vi "RSZVB Set Virtual Transform Port Pair.vi"(0 "VISA session":refnum<visa-resource-name>, 1 "Parameter Type (Capacitance)":i32(ring) items=["Capacitance", "Inductance", "Resistance"], 2 "Circuit Model (Serial Touchstone (.s2p) data, shunt L)":i32(ring)=1 items=["Serial Touchstone (.s2p) data, shunt L"=1, "Serial Touchstone (.s2p) data, shunt C"=2, "Shunt L, serial Touchstone (.s2p) data"=3, "Shunt C, serial Touchstone (.s2p) data"=4, "Serial Cs, shunt L"=5, "Serial Ls, shunt C"=6, "Serial Cs, shunt C"=7, "Serial Ls, shunt L"=8, "Shunt L, serial Cs"=9, "Shunt C, serial Ls"=10, "Shunt C, serial Cs"=11, "Shunt L, serial Ls"=12], 5 "Channel (1)":i32=1, 7 "Function Type (Deembedding)":i32(ring) items=["Deembedding", "Embedding"], 9 "Port Pair (1)":i32=1, 11 "error in (no error)":errorcluster {"code" format="%.0x"}, 12 "Parameter Number (1)":i32=1, 13 "Value (1.0E-12)":dbl=1e-12 format="%^.3e") -> (4 "dup VISA session":refnum<visa-resource-name>, 15 "error out":errorcluster {"code" format="%.0x"})   [LabVIEW 2011]
doc: "This VI specifies the capacitance, inductance or resistance values C1, C2, C3, L1, L2, L3 or R1, R2, R3 in the different circuit models for port pair deembedding/embedding.\n\nRemote-control command(s):\nCALCulate<Ch>:TRANsform:VNETworks:PPAir:DEEMbedding<List_idx>:PARameters:C<no> STSC | SCST | CSSL | LSSC | CSSC | SLCS | SCLS | SCCS,<numeric_value>\nCALCulate<Ch>:TRANsform:VNETworks:PPAir:DEEMbedding<List_idx>:PARameters:L<no> STSL | SLST | CSSL | LSSC | LSSL | SLCS | SCLS | SLLS,<numeric_value>\nCALCulate<Ch>:TRANsform:VNETworks:PPAir:DEEMbedding<List_idx>:PARameters:R<no> STSL | STSC | SLST | SCST | CSSL | LSSC | CSSC | LSSL | SLCS | SCLS | SCCS | SLLS,<numeric_value>\nCALCulate<Ch>:TRANsform:VNETworks:PPAir:EMBedding<List_idx>:PARameters:C<no> STSC | SCST | CSSL | LSSC | CSSC | SLCS | SCLS | SCCS,<numeric_value>\nCALCulate<Ch>:TRANsform:VNETworks:PPAir:EMBedding<List_idx>:PARameters:L<no> STSL | SLST | CSSL | LSSC | LSSL | SLCS | SCLS | SLLS,<numeric_value>\nCALCulate<Ch>:TRANsform:VNETworks:PPAir:EMBedding<List_idx>:PARameters:R<no> STSL | STSC | SLST | SCST | CSSL | LSSC | CSSC | LSSL | SLCS | SCLS | SCCS | SLLS,<numeric_value>"
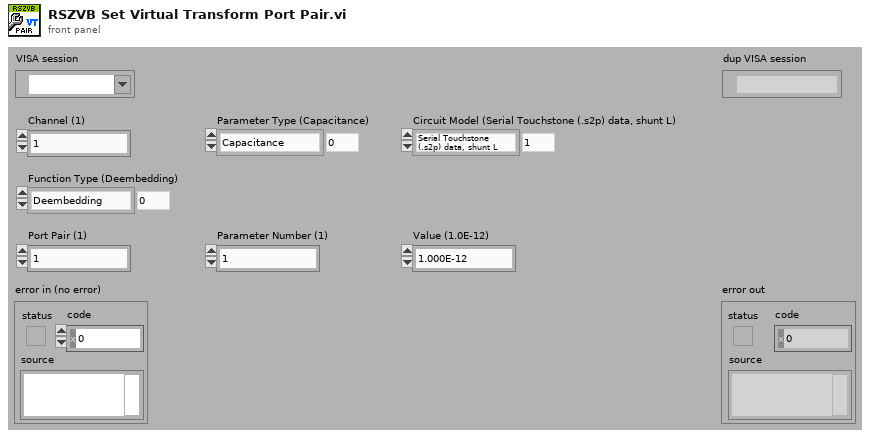
[diagram p1: front panel]
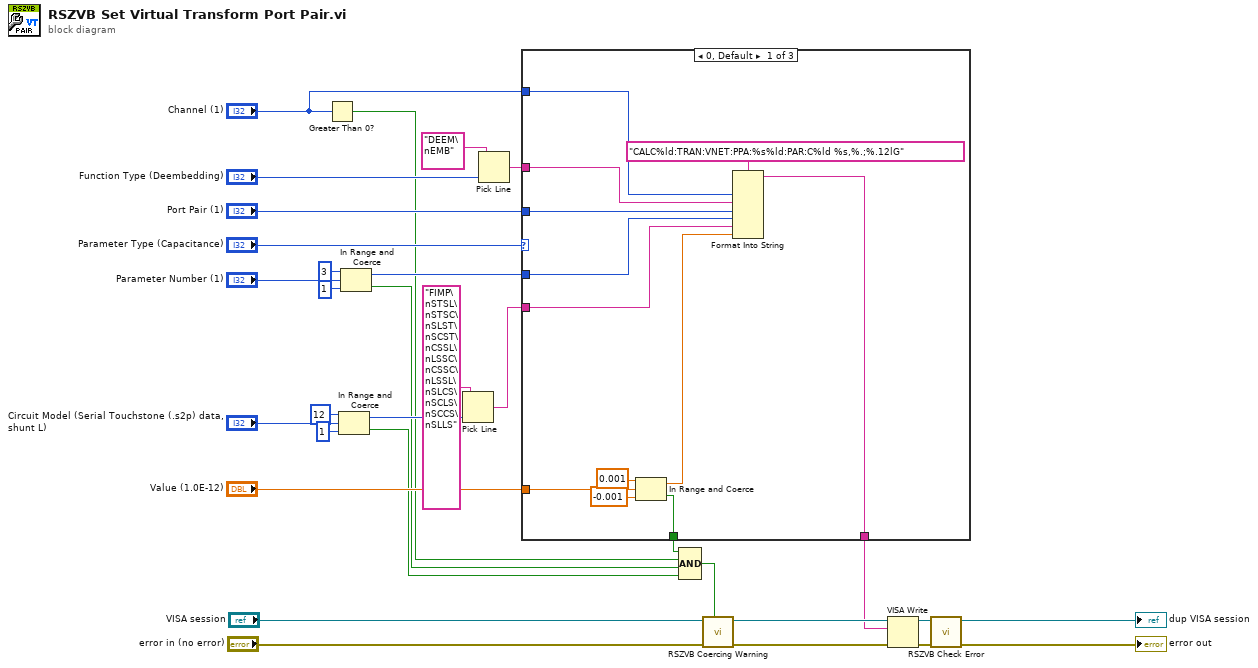
[diagram p0: block diagram]
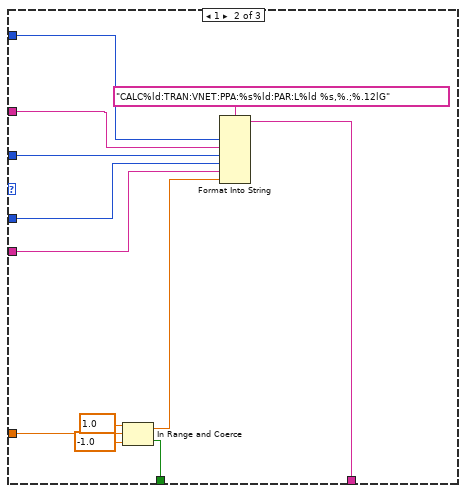
[diagram p2: hidden frame]
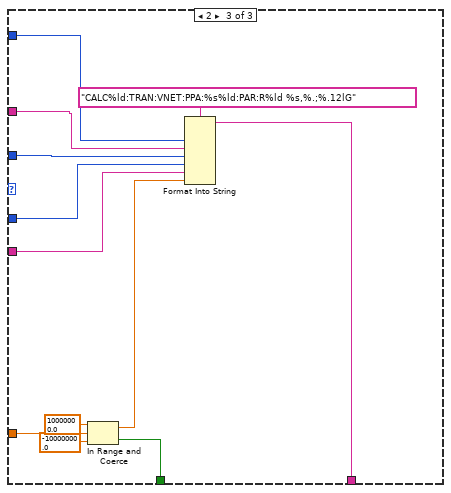
[diagram p3: hidden frame]
diagram:
  n1 = Greater Than 0?(x="Channel (1)") -> (x > 0?=w3:bool)
  n2 = In Range and Coerce(upper limit=12, x="Circuit Model (Serial Touchstone (.s2p) data, shunt L)", lower limit=1) -> (coerced(x)=w7:i32, In Range?=w5:bool)
  n3 = In Range and Coerce(upper limit=3, x="Parameter Number (1)", lower limit=1) -> (coerced(x)=w18:i32, In Range?=w4:bool)
  n4 = Pick Line(multi-line string="FIMP\nSTSL\nSTSC\nSLST\nSCST\nCSSL\nLSSC\nCSSC\nLSSL\nSLCS\nSCLS\nSCCS\nSLLS", line index=w7) -> (output string=w1:string)  [unwired: 1 in]
  n5 = Pick Line(multi-line string="DEEM\nEMB", line index="Function Type (Deembedding)") -> (output string=w23:string)  [unwired: 1 in]
  n6 = case shown="0, Default" "Parameter Type (Capacitance)" {
    tunnel: "Channel (1)" -> [w42 w51 w63]
    tunnel: w23 -> [w41 w50 w62]
    tunnel: "Port Pair (1)" -> [w40 w49 w61]
    tunnel: w18 -> [w39 w48 w60]
    tunnel: [w38 w44 w56] -> w13
    tunnel: "Value (1.0E-12)" -> [w35 w47 w58]
    tunnel: [w33 w46 w57] -> w2
    tunnel: w1 -> [w32 w45 w59]
    frame 0, Default {
      n7 = In Range and Coerce(upper limit=0.001, x=w35, lower limit=-0.001) -> (coerced(x)=w34:dbl, In Range?=w33:bool)
      n8 = Format Into String(format string="CALC%ld:TRAN:VNET:PPA:%s%ld:PAR:C%ld %s,%.;%.12lG", w42, w41, w40, w39, w32, w34) -> (resulting string=w38:string)  [unwired: 2 in, 1 out]
    }
    frame 1 {
      n9 = In Range and Coerce(upper limit=1.0, x=w47, lower limit=-1.0) -> (coerced(x)=w52:dbl, In Range?=w46:bool)
      n10 = Format Into String(format string="CALC%ld:TRAN:VNET:PPA:%s%ld:PAR:L%ld %s,%.;%.12lG", w51, w50, w49, w48, w45, w52) -> (resulting string=w44:string)  [unwired: 2 in, 1 out]
    }
    frame 2 {
      n11 = In Range and Coerce(upper limit=10000000.0, x=w58, lower limit=-10000000.0) -> (coerced(x)=w64:dbl, In Range?=w57:bool)
      n12 = Format Into String(format string="CALC%ld:TRAN:VNET:PPA:%s%ld:PAR:R%ld %s,%.;%.12lG", w63, w62, w61, w60, w59, w64) -> (resulting string=w56:string)  [unwired: 2 in, 1 out]
    }
  }
  n13 = Compound Arithmetic op=AND(w2, w3, w4, w5) -> (w8:bool)
  n14 = call "RSZVB Coercing Warning.vi"("In Range?"=w8, "error in (no error)"="error in (no error)", "VISA session"="VISA session") -> ("error out"=w28:errorcluster, "dup VISA session"=w29:refnum<visa-resource-name>)  [unwired: 7 in]
  n15 = VISA Write(VISA resource name=w29, write buffer=w13, error in (no error)=w28) -> (VISA resource name out=w31:refnum<visa-resource-name>, error out=w30:errorcluster)  [unwired: 1 out]
  n16 = call "RSZVB Check Error.vi"("error in (no error)"=w30, "VISA session"=w31) -> ("error out"=→"error out":errorcluster, "dup VISA session"=→"dup VISA session":refnum<visa-resource-name>)  [unwired: 8 in]
